vi "BRig_Host_dataRunState_dataTS_iSelection.vi"() -> (2 "output_idx_dataTS_iSelection":i32)   [LabVIEW 2014]
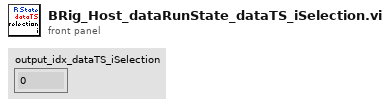
[diagram p1: front panel]
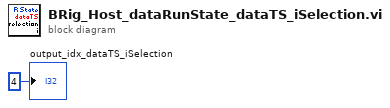
[diagram p0: block diagram]
diagram:
  "output_idx_dataTS_iSelection" <- 4 ("output_idx_dataTS")
